vi "create_random_string.vi"(8 "error in (no error)":errorcluster, 11 "length":i32=14) -> (0 "error out":errorcluster, 3 "random string":string)   [LabVIEW 2010]
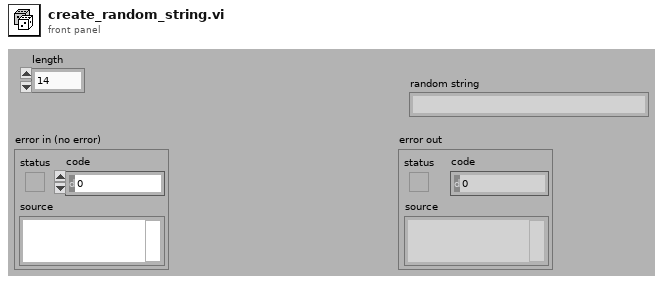
[diagram p1: front panel]
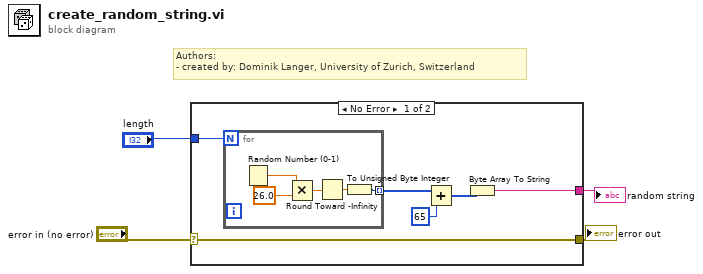
[diagram p0: block diagram]
diagram:
  # "Authors: \n- created by: Dominik Langer, University of Zurich, Switzerland"
  n1 = case shown="No Error" "error in (no error)" {
    selector: "error in (no error)" -> [w10 w16]
    tunnel: [w10 w16] -> w3
    tunnel: [w9 _] -> w2
    tunnel: "length" -> [w8 _]
    frame No Error {
      n2 = for {
        N: w8 -> [_]
        tunnel: [w13] -> w7 mode=indexing
        n3 = Random Number (0-1)() -> (number: 0 to 1=w15:dbl)
        n4 = Multiply(x=w15, y=26.0) -> (x*y=w12:dbl)
        n5 = Round Toward -Infinity(1:w12) -> (0:w11:dbl)
        n6 = To Unsigned Byte Integer(number=w11) -> (unsigned 8bit integer=w13:u8)
      }
      n7 = Add(x=w7, y=u8 65) -> (x+y=w6:u8[])
      n8 = Byte Array To String(unsigned byte array=w6) -> (string=w9:string)
    }
    frame Error {
    }
  }
  "error out" <- w3
  "random string" <- w2
